vi "Listen.vi"(6 "timeout ms (100) (wait forever: -1)":i32=100, 8 "error in (no error)":errorcluster, 11 "RemoteControl.STM in":refnum<class "RemoteControl.STM.lvclass">) -> (0 "error out":errorcluster, 3 "RemoteControl.STM out":refnum<class "RemoteControl.STM.lvclass">)   [LabVIEW 2019, in "RemoteControl.STM.lvclass"]
uses:
  RemoteControl.STM.lvclass
  RemoteControl.STM.lvclass/RemoteControl.STM.ctl
  <vilib>/NI/STM/Connection Manager/TCP/TCP Connection Method.ctl
  <vilib>/NI/STM/TCP/Write Meta Data (TCP Ref).vi
  <vilib>/NI/STM/TCP/Write Meta Data (TCP Clst).vi
  <vilib>/NI/STM/NI STM.lvlib
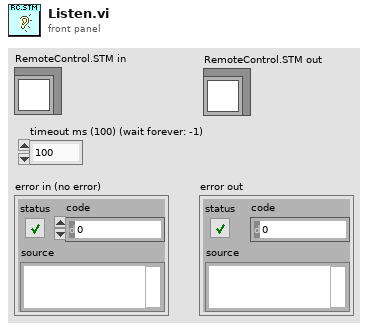
[diagram p1: front panel]
types:
  T1 = typedef "NI STM.lvlib/TCP Connection Method.ctl" = enum16{"Initialize", "Add Connection", "Set Properties", "Get Connection(s)", "Remove Connection", "Remove All Connections", "Get Connection Count"}
  T2 = typedef "NI STM.lvlib/TCP Connection Info.ctl" = cluster{"connection ID":refnum<k5>, "meta data":T3[]}
  T3 = typedef "NI STM.lvlib/MetaDataElement.ctl" = string
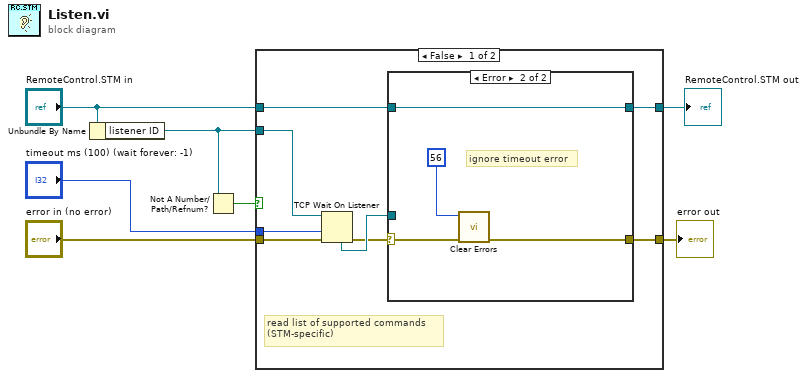
[diagram p0: block diagram]
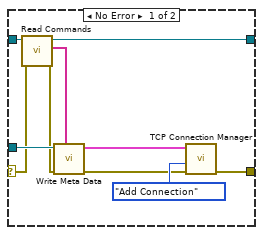
[diagram p2: hidden frame]
diagram:
  n1 = Unbundle By Name("RemoteControl.STM in") -> ("listener ID"=w2:refnum<k5>)
  n2 = Not A Number/Path/Refnum?(number/path/refnum=w2) -> (NaN/Path/Refnum?=w1:bool)
  n3 = case shown="False" w1 {
    tunnel: "error in (no error)" -> [w15 w31]
    tunnel: "RemoteControl.STM in" -> [w9 w30]
    tunnel: [w13 w31] -> w5
    tunnel: [w12 w30] -> w4
    tunnel: "timeout ms (100) (wait forever: -1)" -> [w11 _]
    tunnel: w2 -> [w10 _]
    frame False {
      # "read list of supported commands\n(STM-specific)"
      n4 = TCP Wait On Listener(8:w15, 9:w11, 11:w10) -> (0:w8:errorcluster, 4:w14:refnum<k5>)  [unwired: 1 in, 3 out]
      n5 = case shown="Error" w8 {
        selector: w8 -> [w17 w27]
        tunnel: w14 -> [w25 _]
        tunnel: [w22 w26] -> w13
        tunnel: [w18 w29] -> w12
        tunnel: w9 -> [w20 w29]
        frame No Error {
          n6 = call-dynamic "Read Commands.vi"("error in (no error)"=w17, "RemoteControl in"=w20) -> ("error out"=w16:errorcluster, "Commands"=w19:string[], "RemoteControl out"=w18:refnum<class "RemoteControl.STM.lvclass">)  [unwired: 7 in]
          n7 = call-poly <vilib>:"Write Meta Data.vi"("meta data"=w19, "error in"=w16, "connection ID"=w25) -> ("error out"=w23:errorcluster, "connection info out"=w21:T2)  [unwired: 7 in]
          n8 = call <vilib>:"TCP Connection Manager.vi"("error in"=w23, "method"=TCP_Connection_Method."Add Connection", "connection in"=w21) -> ("error out"=w22:errorcluster)  [unwired: 3 in, 5 out]
        }
        frame Error {
          # "ignore timeout error"
          n9 = call <vilib>:"Clear Errors.vi"("error in (no error)"=w27, "specific error code to clear (0: all)"=56 ("error code")) -> ("error out"=w26:errorcluster)  [unwired: 4 in, 1 out]
        }
      }
    }
    frame True {
    }
  }
  "error out" <- w5
  "RemoteControl.STM out" <- w4
